vi "LunchTest.vi"(8 "error in (no error)":errorcluster, 11 "TestBench in":refnum<class "TestBench.lvclass">) -> (0 "error out":errorcluster, 3 "TestBench out":refnum<class "TestBench.lvclass">)   [LabVIEW 2019, in "TestBench.lvlib" / "TestBench.lvclass"]
uses:
  TestBench.lvclass
  TestBench.lvclass/TestBench.ctl
  <vilib>/ActorFramework/Message Enqueuer/Message Enqueuer.lvclass/Message Enqueuer.ctl
  45fdcf7d-3ff3-4261-87ca-db62d7ee8c67.vi
  <vilib>/ActorFramework/Message Enqueuer/Enqueue.vi
  SystemSetup/SystemSetup Messages/RefreshSystemConfigurationUI Msg/RefreshSystemConfigurationUI Msg.lvclass
  C:/Program Files (x86)/National Instruments/LabVIEW 2019/vi.lib/ActorFramework/Message/Message.lvclass
  <vilib>/ActorFramework/Message Priority Queue/Priority Enqueue.vi
  Assert/Assert.lvlib
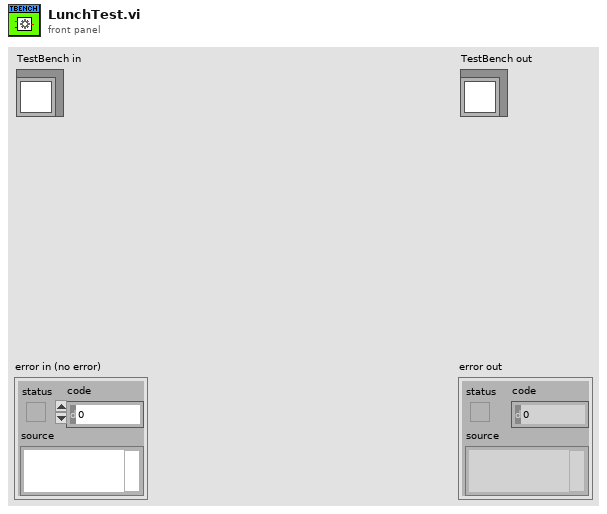
[diagram p1: front panel]
types:
  T1 = enum8{"Enabled", "Disabled", "Disabled and Grayed Out"}
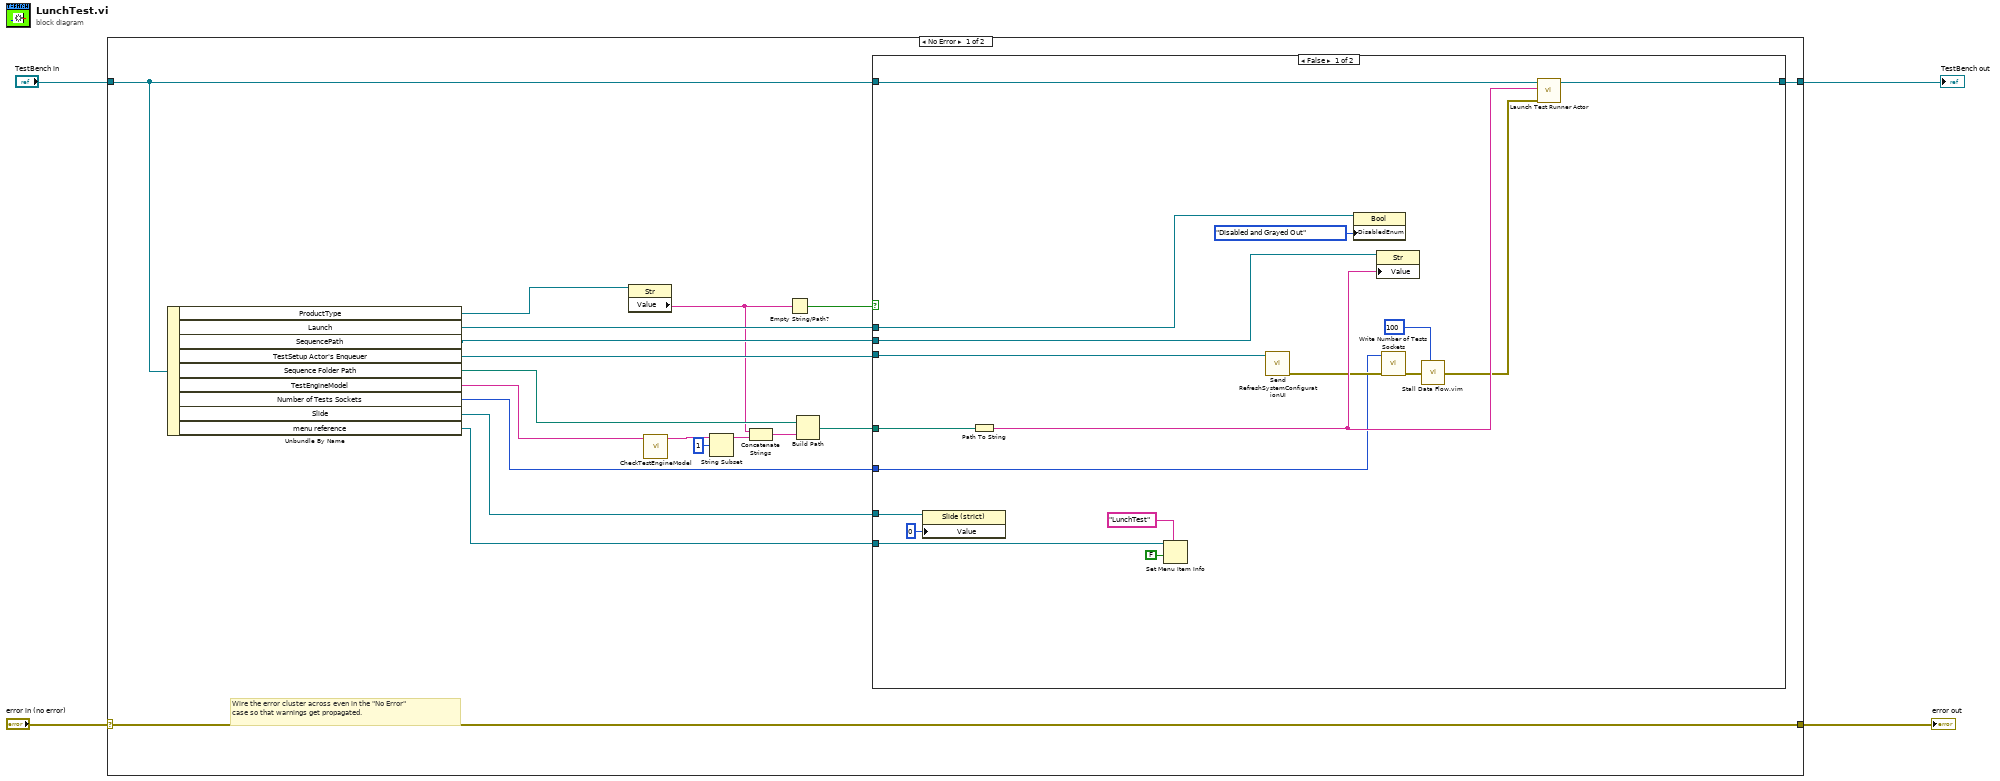
[diagram p0: block diagram]
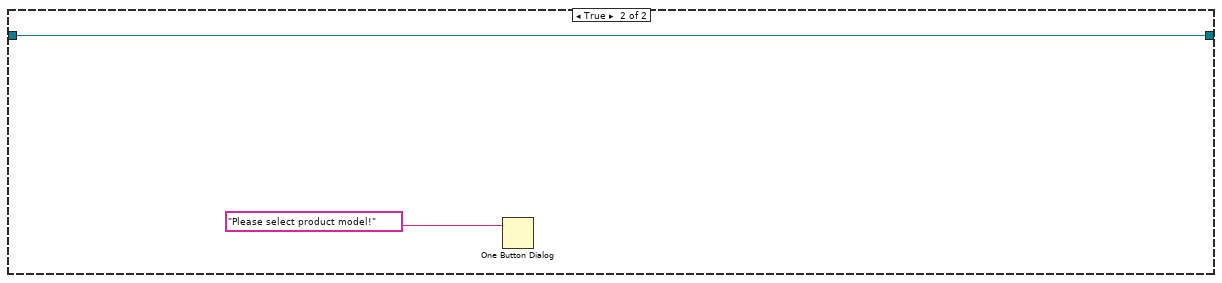
[diagram p2: hidden frame]
diagram:
  n1 = case shown="No Error" "error in (no error)" {
    selector: "error in (no error)" -> [w23 w45]
    tunnel: [w23 w45] -> w3
    tunnel: [w5 w44] -> w1
    tunnel: "TestBench in" -> [w6 w44]
    frame No Error {
      # "Wire the error cluster across even in the \"No Error\"\ncase so that warnings get propagated."
      n2 = Unbundle By Name(w6) -> ("ProductType"=w7:refnum<vi>, "Launch"=w18:refnum<vi>, "SequencePath"=w19:refnum<vi>, "TestSetup Actor's Enqueuer"=w22:refnum<class "Message Enqueuer.lvclass">, "Sequence Folder Path"=w17:path, "TestEngineModel"=w13:string, "Number of Tests Sockets"=w20:u8, "Slide"=w9:refnum<vi>, "menu reference"=w8:refnum<k9>)
      n3 = property class="Str"(reference=w7) -> ("Value"=w15:string)  [unwired: 1 in, 2 out]
      n4 = call "CheckTestEngineModel.vi"("Modle"=w13) -> ("Pattern"=w12:string)  [unwired: 10 in]
      n5 = String Subset(string=w12, offset (0)=1) -> (substring=w11:string)  [unwired: 1 in]
      n6 = Concatenate Strings(w15, w11) -> (w16:string)
      n7 = Empty String/Path?(string/path=w15) -> (empty?=w21:bool)
      n8 = Build Path(base path=w17, name or relative path=w16) -> (appended path=w14:path)
      n9 = case shown="False" w21 {
        tunnel: w22 -> [w41 _]
        tunnel: w19 -> [w40 _]
        tunnel: w20 -> [w24 _]
        tunnel: w18 -> [w39 _]
        tunnel: w14 -> [w38 _]
        tunnel: w9 -> [w37 _]
        tunnel: w8 -> [w36 _]
        tunnel: w6 -> [w30 w42]
        tunnel: [w29 w42] -> w5
        frame False {
          n10 = property class="Slide (strict)"(reference=w37, "Value"=u32 0) -> ()  [unwired: 1 in, 2 out]
          n11 = Path To String(path=w38) -> (string=w28:string)
          n12 = Set Menu Item Info(7:"LunchTest" ("item tag"), 9:FALSE ("enabled"), 11:w36) -> ()  [unwired: 4 in, 2 out]
          n13 = call "Send RefreshSystemConfigurationUI.vi"("Message Enqueuer"=w41) -> ("error out"=w26:errorcluster)  [unwired: 9 in, 1 out]
          n14 = property class="Bool"(reference=w39, "DisabledEnum"=T1."Disabled and Grayed Out" ("Disabled")) -> ()  [unwired: 1 in, 2 out]
          n15 = property class="Str"(reference=w40, "Value"=w28) -> ()  [unwired: 1 in, 2 out]
          n16 = call "Write Number of Tests Sockets.vi"("error in (no error)"=w26, "Number of Tests Sockets"=w24) -> ("error out"=w25:errorcluster)  [unwired: 9 in]
          n17 = call "Stall Data Flow.vim"("value in"=w25, "milliseconds to wait"=u32 100) -> ("value out"=w27:errorcluster)  [unwired: 1 out]
          n18 = call "Launch Test Runner Actor.vi"("error in (no error)"=w27, "SequncePath"=w28, "TestBench in"=w30) -> ("TestBench out"=w29:refnum<class "TestBench.lvclass">)  [unwired: 7 in, 1 out]
        }
        frame True {
          n19 = One Button Dialog(message="Please select product model!") -> ()  [unwired: 1 in, 1 out]
        }
      }
    }
    frame Error {
    }
  }
  "error out" <- w3
  "TestBench out" <- w1
